vi "Close Data File.vi"(8 "error in (no error)":errorcluster, 11 "DbMeasurement in":refnum<class "DbMeasurement.lvclass">) -> (0 "error out":errorcluster, 3 "DbMeasurement out":refnum<class "DbMeasurement.lvclass">)   [LabVIEW 2013, in "DbMeasurement.lvclass"]
doc: "This static method closes the data file, which points to a database link. This VI executes normally even if an error occurs before hand."
uses:
  DbMeasurement.lvclass
  DbMeasurement.lvclass/DbMeasurement.ctl
  <vilib>/addons/database/NI_Database_API.lvlib
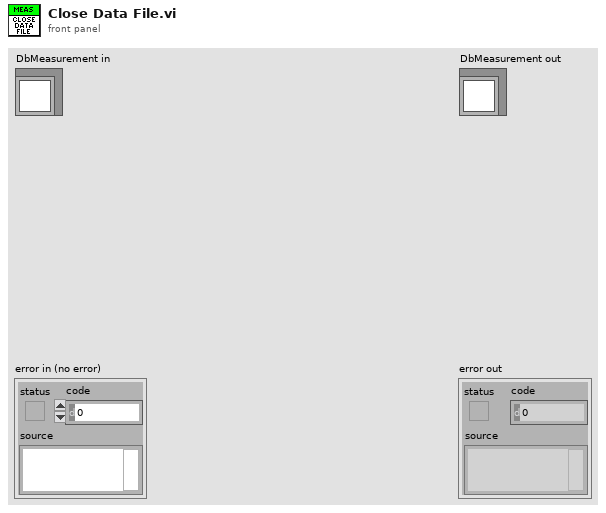
[diagram p1: front panel]
types:
  T1 = typedef "NI_Database_API.lvlib/Conn ObjectReference.ctl" = refnum<k1>
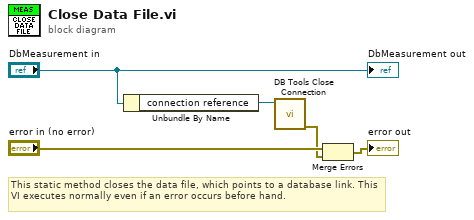
[diagram p0: block diagram]
diagram:
  # "This static method closes the data file, which points to a database link. This VI executes normally even if an error occurs before hand."
  n1 = Unbundle By Name("DbMeasurement in") -> ("connection reference"=w4:T1)
  n2 = call <vilib>:"DB Tools Close Connection.vi"("connection reference"=w4) -> ("error out"=w1:errorcluster)  [unwired: 6 in]
  n3 = Merge Errors("error in (no error)", w1) -> (→"error out":errorcluster)
  "DbMeasurement out" <- "DbMeasurement in"
